vi "Bairstow Root Finding (CDB).vi"(9 "threshold":dbl=0.001, 10 "Conjugate Complex Root Candidates":cdb[](array[numeric]), 11 "P(x)":dbl[](array[numeric])) -> (2 "Complex Roots":cdb[](array[numeric]), 3 "Real Roots":dbl[](array[numeric]))   [LabVIEW 2010, in "NI_AALPro.lvlib"]
uses:
  NI_AALPro.lvlib
  Create Polynomial From Roots (CDB).vi
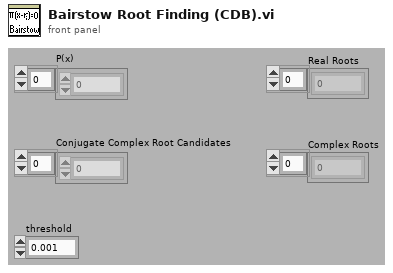
[diagram p1: front panel]
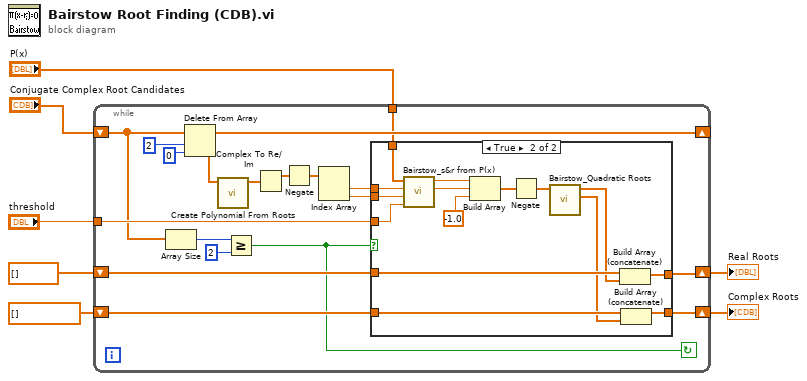
[diagram p0: block diagram]
diagram:
  n1 = while {
    tunnel: "threshold" -> [w26]
    shift-right: [w24] -> w2
    shift-left: dbl[] [] -> [w25]
    shift-right: [w22] -> w1
    shift-left: cdb[] [] -> [w23]
    shift-right: [w15] -> _
    shift-left: "Conjugate Complex Root Candidates" -> [w17]
    tunnel: "P(x)" -> [w8]
    stop <- w18 continue-if-true
    n2 = Array Size(array=w17) -> (size(s)=w20:i32)
    n3 = Delete From Array(array=w17, length=2, index=0) -> (deleted portion=w14:cdb[], array with subset deleted=w15:cdb[])
    n4 = call-poly "Create Polynomial From Roots.vi"("Roots"=w14) -> ("P(x)"=w16:cdb[])  [unwired: 9 in, 1 out]
    n5 = Greater Or Equal?(x=w20, y=2) -> (x >= y?=w18:bool)
    n6 = Complex To Re/Im(x + iy=w16) -> (x=w12:dbl[])  [unwired: 1 out]
    n7 = Negate(x=w12) -> (-x=w11:dbl[])
    n8 = Index Array(array=w11) -> (element #1=w10:dbl, element #2=w9:dbl)  [unwired: 2 in]
    n9 = case shown="True" w18 {
      tunnel: w26 -> [_ w43]
      tunnel: w25 -> [w28 w41]
      tunnel: [w28 w40] -> w24
      tunnel: w23 -> [w27 w38]
      tunnel: [w27 w36] -> w22
      tunnel: w10 -> [_ w31]
      tunnel: w9 -> [_ w30]
      tunnel: w8 -> [_ w29]
      frame False {
      }
      frame True {
        n10 = call "Bairstow_s&r from P(x).vi"("threshold"=w43, "r in"=w30, "s in"=w31, "P(x)"=w29) -> ("r out"=w34:dbl, "s out"=w35:dbl)  [unwired: 6 in]
        n11 = Build Array(w35, w34, -1.0 ("y")) -> (w32:dbl[])
        n12 = Negate(x=w32) -> (-x=w33:dbl[])
        n13 = call "Bairstow_Quadratic Roots.vi"("quadratic"=w33) -> ("Complex Pair Roots"=w37:cdb[], "Real Roots"=w39:dbl[])  [unwired: 9 in]
        n14 = Build Array (concatenate)(w41, w39) -> (w40:dbl[])
        n15 = Build Array (concatenate)(w38, w37) -> (w36:cdb[])
      }
    }
  }
  "Real Roots" <- w2
  "Complex Roots" <- w1
